vi "Init Msg.vi"(6 "Teller":refnum<class "Teller.lvclass">, 9 "Error":errorcluster, 10 "Unified Actor":refnum<class "Actor.lvclass">) -> (2 "Msg":refnum<class "Msg.lvclass">)   [LabVIEW 2020, in "jettl.lvlib" / "Stopped jettl Msg.lvlib" / "Stopped.lvlib"]
uses:
  Stopped.lvlib
  Teller/Teller.lvclass
  Msg/Msg.lvclass
  Actor/Actor.lvclass
  Stopped Msg Input/Stopped Msg Input.lvlib
  Stopped Msg/Stopped Msg.lvlib
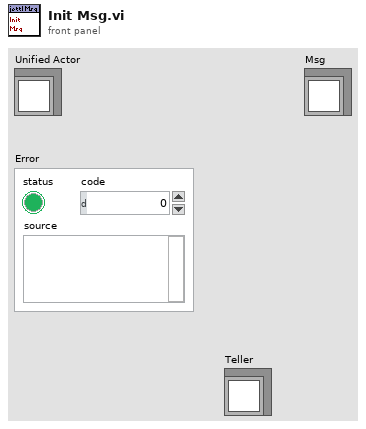
[diagram p1: front panel]
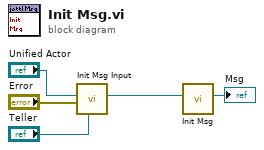
[diagram p0: block diagram]
diagram:
  n1 = call "Init Msg Input.vi"("Teller"="Teller", "Error"="Error", "Unified Actor"="Unified Actor") -> ("Msg Input"=w5:refnum<class "Msg Input.lvclass">)  [unwired: 8 in]
  n2 = call "Init Msg.vi"("Msg Input"=w5) -> ("Msg"=→"Msg":refnum<class "Msg.lvclass">)  [unwired: 10 in]
